vi "Logger.Variant.UpdateSerialNo.vi"() -> ()   [LabVIEW 2016]
panel:
  in  "FilePath 2":path=path "D:/Maszup/WABCO/SVN/LaserMarkingStation/SOFTWARE/settings/Variants11.ini"
  out "min value 2":i32
  out "min value":i32
  out "element":i32
  in  "FilePath":path=path "D:/Maszup/WABCO/SVN/LaserMarkingStation/SOFTWARE/settings/Variants1.ini"
  out "sum":i16
  in  "All":i32(listbox)
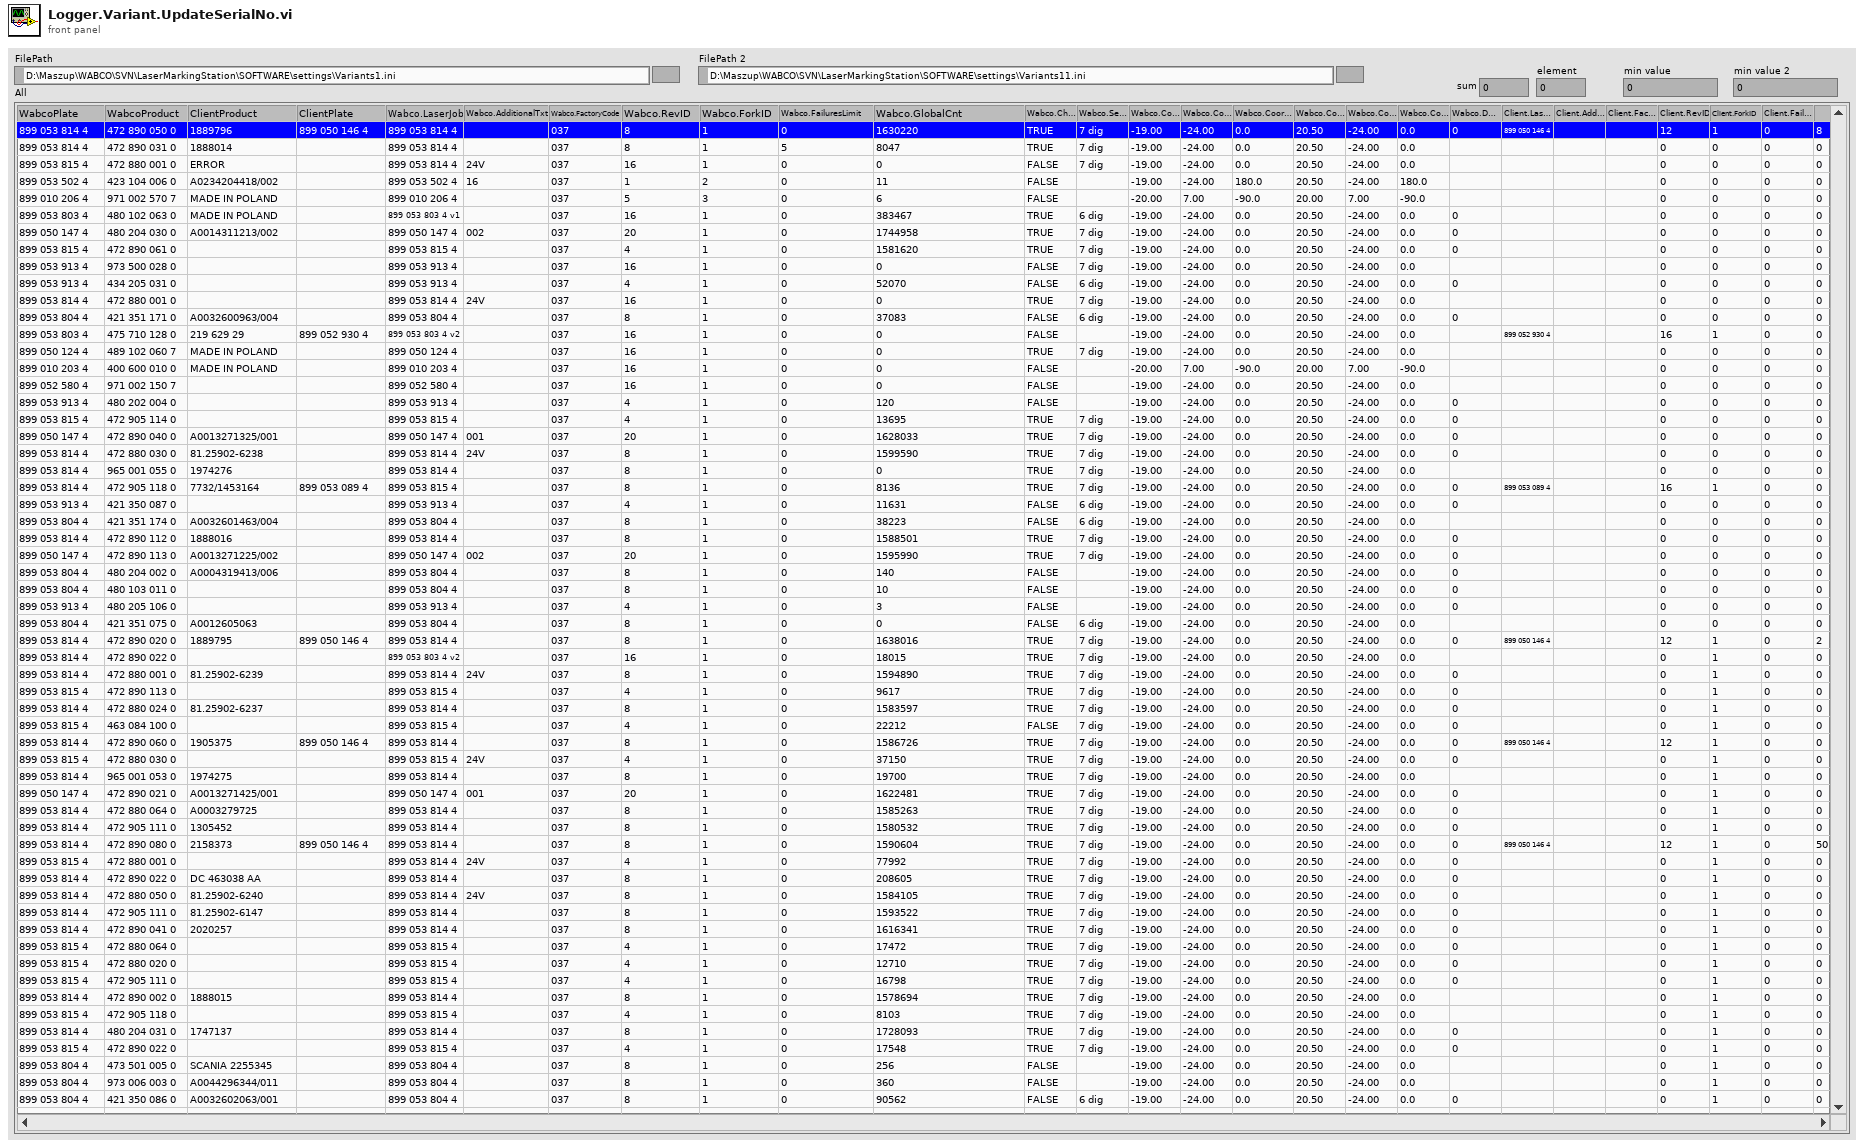
[diagram p1: front panel]
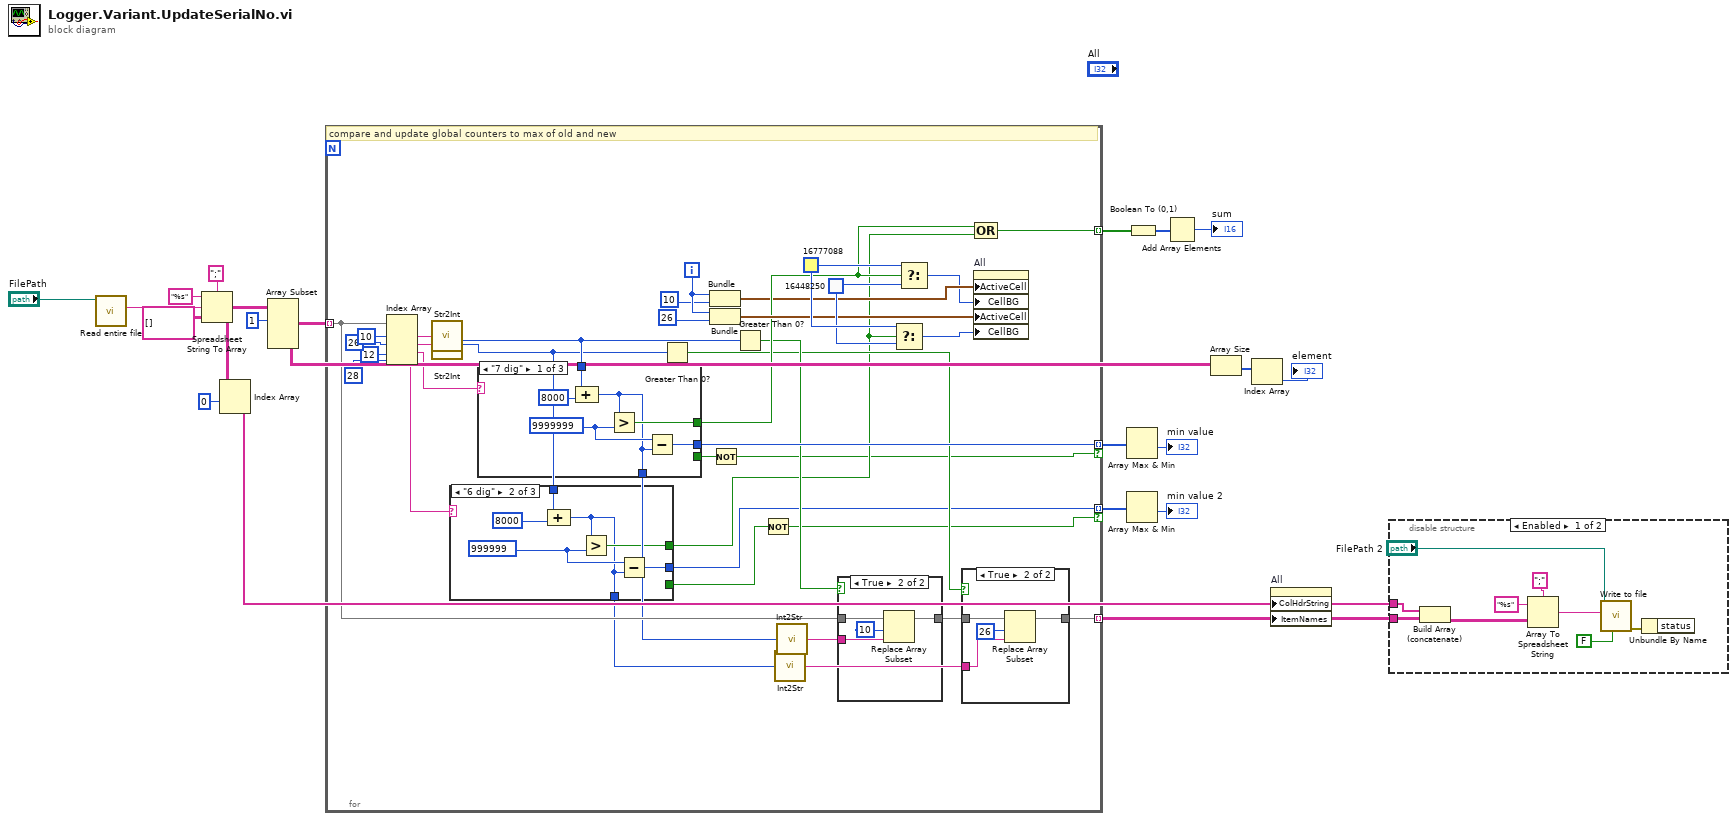
[diagram p0: block diagram]
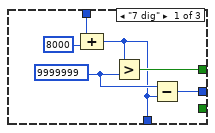
[diagram p3: hidden frame]
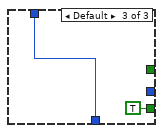
[diagram p4: hidden frame]
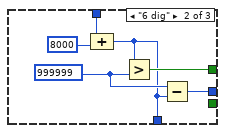
[diagram p7: hidden frame]
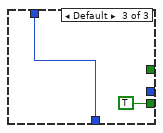
[diagram p8: hidden frame]
diagram:
  n1 = call "Read entire file.vi"("file"="FilePath") -> ("contents"=w20:string)  [unwired: 5 in, 1 out]
  n2 = Spreadsheet String To Array(delimiter (Tab)=";", format string="%s", spreadsheet string=w20, array type (2D Dbl)=string[][] []) -> (array=w11:string[][])
  n3 = Index Array(array=w11, index (row)=0) -> (element=w9:string[])  [unwired: 1 in]
  n4 = Array Subset(array=w11, index (row)=1 ("index")) -> (w8:string[][])  [unwired: 3 in]
  n5 = for {
    tunnel: w8 -> [w38] mode=indexing
    tunnel: [w56] -> w15 mode=indexing
    tunnel: [w44] -> w5 mode=indexing if=w25
    tunnel: [w27] -> w4 mode=indexing if=w24
    tunnel: [w35] -> w1 mode=indexing
    i -> [w57]
    w53 = u32 16448250
    w54 = u32 16777088
    # "compare and update global counters to max of old and new"
    n6 = Index Array(array=w38, index #1=10 ("index"), index #2=26 ("index"), index #3=12 ("index"), index #4=28 ("index")) -> (element #1=w50:string, element #2=w49:string, element #3=w39:string, element #4=w29:string)
    n7 = call "Str2Int.vi"("string"=w50) -> ("Numeric"=w46:i32)
    n8 = call "Str2Int.vi"("string"=w49) -> ("Numeric"=w31:i32)
    n9 = case shown="\"6 dig\"" w29 {
      tunnel: w31 -> [w63 w69 w70]
      tunnel: [w62 w68 _] -> w28
      tunnel: [w59 w65 _] -> w27
      tunnel: [_ _ TRUE] -> w23
      tunnel: [w58 w64 w70] -> w21
      frame "7 dig" {
        w60 = 9999999 ("Numeric")
        n10 = Compound Arithmetic op=ADD(w63, 8000 ("value")) -> (w58:i32)
        n11 = Greater?(x=w58, y=w60) -> (0:w62:bool)
        n12 = Subtract(x=w60, y=w58) -> (x-y=w59:i32)
      }
      frame "6 dig" {
        w66 = 999999 ("Numeric")
        n13 = Compound Arithmetic op=ADD(w69, 8000 ("value")) -> (w64:i32)
        n14 = Greater?(x=w64, y=w66) -> (0:w68:bool)
        n15 = Subtract(x=w66, y=w64) -> (x-y=w65:i32)
      }
      frame Default {
      }
    }
    n16 = case shown="\"7 dig\"" w39 {
      tunnel: w46 -> [w87 w93 w94]
      tunnel: [w86 w92 _] -> w45
      tunnel: [w83 w89 _] -> w44
      tunnel: [_ _ TRUE] -> w26
      tunnel: [w82 w88 w94] -> w22
      frame "7 dig" {
        w84 = 9999999 ("Numeric")
        n17 = Compound Arithmetic op=ADD(w87, 8000 ("value")) -> (w82:i32)
        n18 = Greater?(x=w82, y=w84) -> (0:w86:bool)
        n19 = Subtract(x=w84, y=w82) -> (x-y=w83:i32)
      }
      frame "6 dig" {
        w90 = 999999 ("Numeric")
        n20 = Compound Arithmetic op=ADD(w93, 8000 ("value")) -> (w88:i32)
        n21 = Greater?(x=w88, y=w90) -> (0:w92:bool)
        n22 = Subtract(x=w90, y=w88) -> (x-y=w89:i32)
      }
      frame Default {
      }
    }
    n23 = Greater Than 0?(x=w31) -> (x > 0?=w32:bool)
    n24 = Bundle(w57, "index"=10) -> (w41:cluster{i32, "index":i32})  [unwired: 1 in]
    n25 = Bundle(w57, "index"=26) -> (w52:cluster{i32, "index":i32})  [unwired: 1 in]
    n26 = Not(x=w26) -> (.not. x?=w25:bool)
    n27 = Greater Than 0?(x=w46) -> (x > 0?=w33:bool)
    n28 = Not(x=w23) -> (.not. x?=w24:bool)
    n29 = call "Int2Str.vi"("Numeric"=w21) -> ("string"=w34:string)
    n30 = call "Int2Str.vi"("Numeric"=w22) -> ("string"=w37:string)
    n31 = case shown="True" w33 {
      tunnel: w38 -> [w77 w81]
      tunnel: w37 -> [_ w79]
      tunnel: [w77 w78] -> w36
      frame False {
      }
      frame True {
        n32 = Replace Array Subset(array=w81, new element=w79, index=10) -> (w78:string[])
      }
    }
    n33 = Select(t=w54, s=w28, f=w53) -> (s? t:f=w51:u32)
    n34 = Select(t=w54, s=w45, f=w53) -> (s? t:f=w40:u32)
    n35 = case shown="True" w32 {
      tunnel: w36 -> [w72 w76]
      tunnel: [w72 w75] -> w35
      tunnel: w34 -> [_ w73]
      frame False {
      }
      frame True {
        n36 = Replace Array Subset(array=w76, new element=w73, index=26) -> (w75:string[])
      }
    }
    n37 = property on="All" class="MCListbox (strict)"("ActiveCell"=w41, "CellBG"=w40, "ActiveCell"=w52, "CellBG"=w51) -> ()  [unwired: 2 in, 2 out]
    n38 = Compound Arithmetic op=OR(w45, w28) -> (w56:bool)
  }
  n39 = Array Max & Min(array=w5) -> (min value=→"min value":i32)  [unwired: 3 out]
  n40 = Array Max & Min(array=w4) -> (min value=→"min value 2":i32)  [unwired: 3 out]
  n41 = Boolean To (0,1)(Boolean=w15) -> (0, 1=w14:i16[])
  n42 = Add Array Elements(numeric array=w14) -> (sum=→"sum":i16)
  n43 = Array Size(array=w8) -> (size(s)=w7:i32[])
  n44 = Index Array(array=w7) -> (element=→"element":i32)  [unwired: 1 in]
  n45 = property on="All" class="MCListbox (strict)"("ColHdrString"=w9, "ItemNames"=w1) -> ()  [unwired: 2 in, 2 out]
  n46 = disable-structure shown="Enabled" {
    disable-tunnel: w1 -> [w100 _]
    disable-tunnel: w9 -> [w99 _]
    frame Enabled {
      n47 = Build Array (concatenate)(w99, w100) -> (w98:string[][])
      n48 = Array To Spreadsheet String(delimiter (Tab)=";", array=w98, 3:"%s" ("format string")) -> (spreadsheet string=w101:string)
      n49 = call "Write to file.vi"("append (F)"=FALSE, "addition"=w101, "file"="FilePath 2") -> ("error out"=w97:errorcluster)  [unwired: 8 in]
      n50 = Unbundle By Name(w97) -> ()  [unwired: 1 out]
    }
    frame Disabled {
    }
  }
